vi "DEV test VIs Wrapped.vi"(8 "Error In":errorcluster) -> (0 "Error Out":errorcluster)   [LabVIEW 2018, in "Receipt Parsing.lvlib"]
uses:
  Receipt Parsing.lvlib
panel:
  out "data":string
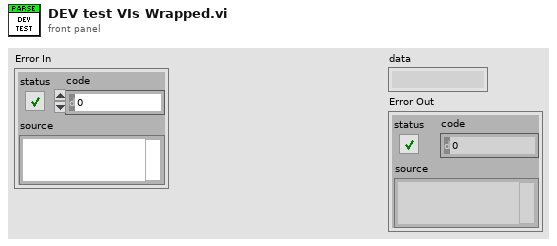
[diagram p1: front panel]
types:
  T1 = typedef "IMAQ Image.ctl" = refnum<image>
  T2 = typedef "ROI Descriptor" = cluster{"Global Rectangle":i32[], "Contours":cluster{"ID":enum32{"External", "Internal"}, "Type":u32, "Coordinates":i32[]}[]}
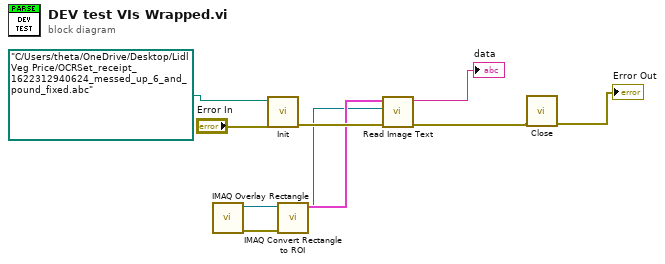
[diagram p0: block diagram]
diagram:
  n1 = call "IMAQ Overlay Rectangle"() -> ("error out"=w6:errorcluster, "Image Out"=w4:T1)  [unwired: 10 in]
  n2 = call "Init.vi"("error in (no error)"="Error In", "File Path"=path "C:/Users/theta/OneDrive/Desktop/Lidl Veg Price/OCRSet_receipt_1622312940624_messed_up_6_and_pound_fixed.abc") -> ("error out"=w7:errorcluster)  [unwired: 9 in]
  n3 = call "IMAQ Convert Rectangle to ROI"("error in (no error)"=w6) -> ("ROI Descriptor"=w5:T2)  [unwired: 8 in, 1 out]
  n4 = call "Read Image Text.vi"("Error In"=w7, "ROI Descriptor"=w4, "Image Ref"=w5) -> ("Error Out"=w3:errorcluster, "Line of Text"=→"data":string)  [unwired: 7 in]
  n5 = call "Close.vi"("error in (no error)"=w3) -> ("error out"=→"Error Out":errorcluster)  [unwired: 10 in]
